vi "SE_HV500.SetVoltage.vi"(0 "i ref in":refnum<vi>, 2 "Set Voltage":dbl format="%.5f", 3 "Channel":i16, 4 "Time out":i32, 5 "error in (no error)":errorcluster) -> (14 "i ref out":refnum<vi>, 16 "timed out":bool, 19 "error out":errorcluster)   [LabVIEW 2014, in "SE_HV500.lvlib"]
doc: "Sets the Voltage at the Device. but first one should increase the current to set the voltage else the Voltage might not be set"
uses:
  SE_HV500.lvlib
  CS_Core/CSSystem/CoreDefs/CoreDefs.error_type.ctl
  CS_Core/CSSystem/CoreLib/CoreLib.lvlib
  instr.lib/SE_HV500_Driver/SE_HV500Driver.lvlib
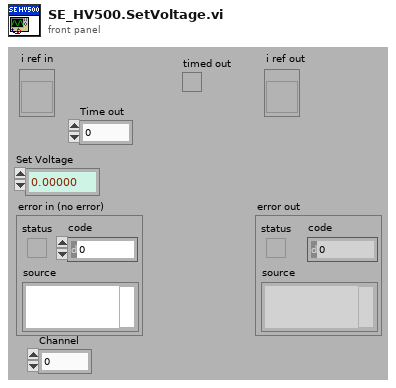
[diagram p1: front panel]
types:
  T1 = typedef "CoreDefs.error_type.ctl" = enum16{"no error", "can't load process", "can't unload process", "process does not exist", "can't install process", "can't remove process", "unknown function", "time out", "can't execute function", "duplicate queue name", "super not found", "caller queue invalid", "can't ping process", "unknown error", "VISA Error", "VISA timeout", "GPIB timeout", "GPIB error", "communication error", "data type mismatch", "can't read data from OPC server", "can't write data to OPC server", "OET error", "function not implemented", "process already exists", "invalid Shared Variable name", "error writing Shared Variable", "error reading Shared Variable", "invalid client name", "corrupt database", "unknown class", "call not authorized", "parameter out of range", "OET timeout: can't get data to modify", "invalid queue name", "requested operation incompatible with current state", "event undefined", "event disabled", "state undefined", "caller is not a friend", "EventBuilder: bad eventID", "EventBuilder: no DAQ devices", "a thread must not stop itself", "UNUSED ELEMENT4", "DiscArchiver: eventData incomplete", "DiscArchiver: eventData does not belong to run", "DiscArchiver: can't open file", "DiscArchiver: can't write to file", "DiscArchiver: available disc space low", "can't acquire semaphore", "error reading data from database", "notifier object is not existing", "can't register process", "can't unregister process", "illegal event type", "object disabled", "object already exists", "can't change state", "Instrument not found", "no connection to remote node", "invalid reference", "N/A", "UNUSED ELEMENT 1", "element not found", "illegal TCP/IP connection detected", "object does not exist", "invalid access ID", "unknown CS system", "invalid privilige", "unsupported data type", "unsupported server type", "IO server already exists", "Shared Variable already exists"}
  T2 = typedef "SE_HV500.lvlib/SE_HV500.i attribute.ctl" = cluster{"SetStatus":bool, "Set Voltage":dbl, "VoltageID":i32, "Nom Voltage":dbl, "VISA resource name in":refnum<visa-resource-name>, "Device name":string, "PSRange":i32}
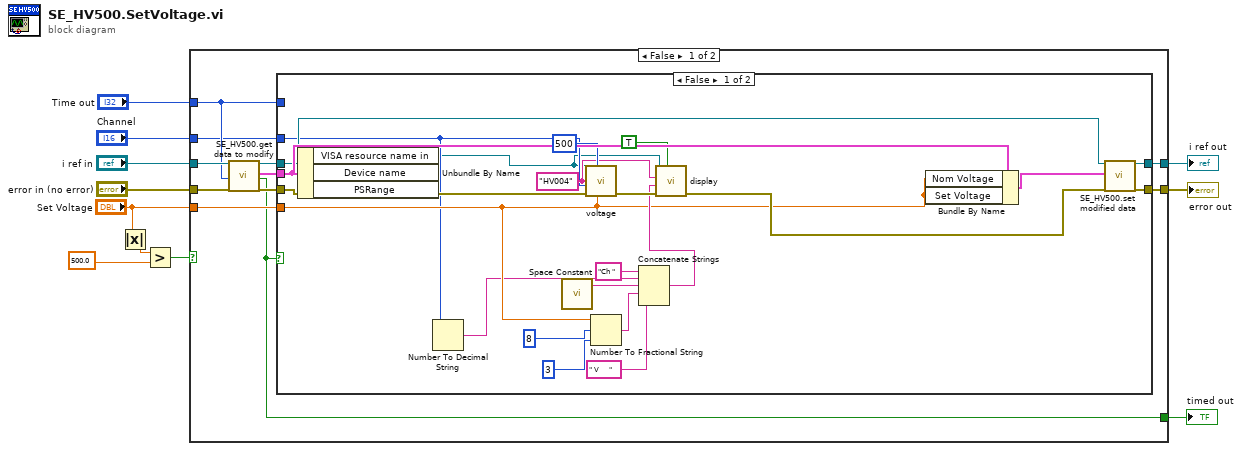
[diagram p0: block diagram]
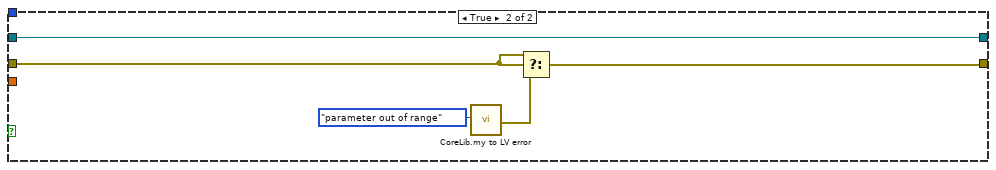
[diagram p3: hidden frame]
diagram:
  n1 = Absolute Value(x="Set Voltage") -> (abs(x)=w2:dbl)
  n2 = Greater?(x=w2, y=500.0) -> (0:w6:bool)
  n3 = case shown="False" w6 {
    tunnel: [w22 w47] -> w11
    tunnel: "Set Voltage" -> [w21 _]
    tunnel: [w20 w51] -> w10
    tunnel: "i ref in" -> [w18 w51]
    tunnel: "error in (no error)" -> [w16 w49]
    tunnel: "Time out" -> [w17 _]
    tunnel: [w13 _] -> w5
    tunnel: "Channel" -> [w12 _]
    frame False {
      n4 = call "SE_HV500.get data to modify.vi"("i ref in"=w18, "ms timeout (10000)"=w17, "error in (no error)"=w16) -> ("i ref out"=w19:refnum<vi>, "i attribute"=w14:T2, "timed out"=w13:bool, "error out"=w15:errorcluster)  [unwired: 13 in]
      n5 = case shown="False" w13 {
        tunnel: w14 -> [w41 _]
        tunnel: w15 -> [w42 w45]
        tunnel: [w43 w45] -> w22
        tunnel: w21 -> [w28 _]
        tunnel: w19 -> [w39 w46]
        tunnel: [w44 w46] -> w20
        tunnel: w17 -> [_ _]
        tunnel: w12 -> [w25 _]
        frame False {
          w30 = "HV004" ("Device name")
          n6 = Unbundle By Name(w41) -> ("VISA resource name in"=w23:refnum<visa-resource-name>)  [unwired: 2 out]
          n7 = Number To Decimal String(number=w25) -> (decimal integer string=w26:string)  [unwired: 1 in]
          n8 = call <vilib>:"Space Constant.vi"() -> ("String"=w24:string)
          n9 = call "voltage.vi"("Voltage"=w28, "Span"=500, "Error in"=w42, "Channel nr."=w25, "Device name"=w30, "VISA resource name in"=w23) -> ("Error out"=w33:errorcluster)  [unwired: 3 in, 2 out]
          n10 = Number To Fractional String(number=w28, width (-)=8, precision (6)=3) -> (F-format string=w37:string)  [unwired: 1 in]
          n11 = Concatenate Strings("Ch " ("string"), w26, w24, w37, " V     " ("string")) -> (w31:string)
          n12 = call "display.vi"("Next free line"=TRUE, "Error in"=w33, "Display String"=w31, "Device name"=w30, "VISA resource name in"=w23) -> ("Error out"=w32:errorcluster)  [unwired: 5 in, 1 out]
          n13 = Bundle By Name(cluster=w41, "Nom Voltage"=w28, "Set Voltage"=w28) -> (w40:T2)
          n14 = call "SE_HV500.set modified data.vi"("i ref in"=w39, "i attribute"=w40, "error in (no error)"=w32) -> ("i ref out"=w44:refnum<vi>, "error out"=w43:errorcluster)  [unwired: 15 in]
        }
        frame True {
        }
      }
    }
    frame True {
      n15 = call "CoreLib.my to LV error.vi"("ErrorTypes"=CoreDefs.error_type."parameter out of range") -> ("myErrorCluster"=w48:errorcluster)  [unwired: 17 in, 1 out]
      n16 = Select(t=w49, s=w49, f=w48) -> (s? t:f=w47:errorcluster)
    }
  }
  "error out" <- w11
  "i ref out" <- w10
  "timed out" <- w5
